vi "sql-readinfo-fixture.vi"(0 "input-IP":string="dg-sql-01.luxshare.com.cn", 1 "input-user":string="htpsuser", 3 "input-psw":string="htps'songyy", 4 "input-db":string="HTPSDB", 5 "操作模式":T1(ring)=enum."查询数据", 7 "查询项目":string="LuxsharePN,CustomerPN,Customer,SampleDes,AWG,Length,EEPROMWrite,LabelPrint,Remarks", 8 "表名":string="vfixture", 11 "标识列":string, 12 "限定条件":string="where LuxsharePN='L12345678'", 13 "Page":string, 15 "Desc":string) -> (14 "数据输出2":dbl[][](array[numeric]), 16 "错误类型":string, 17 "StringArray2":string[][](array[string])=[["L12345678\t\tIBM\t40G Ethernet QSFP+ Passive DAC Cable\t28\t3000\t0\t0\trefer to IBM Spec"]], 18 "列内对数":i32=1, 19 "返回记录数目":i32=1, 20 "ConvertToArray":string[][](array[string])=[["L12345678", "", "IBM", "40G Ethernet QSFP+ Passive DAC Cable", "28", "3000", "0", "0", "refer to IBM Spec"]], 21 "status":bool, 23 "ResultString":string="L12345678\t\tIBM\t40G Ethernet QSFP+ Passive DAC Cable\t28\t3000\t0\t0\trefer to IBM Spec\r", 24 "ConvertToClusterArray":cluster{"项":string, "值":string}[](array[cluster])=[{"项"="", "值"=""}, {"项"="L12345678", "值"="L12345678"}], 25 "DataPair":dbl[](array[numeric]), 27 "数据输出":dbl[][](array[numeric]))   [LabVIEW 2011]
panel:
  out "result string":string="select LuxsharePN,CustomerPN,Customer,SampleDes,AWG,Length,EEPROMWrite,LabelPrint,Remarks from project where LuxsharePN='L12345678'"
  out "替换数量":i32=9
  in  "二级分隔符":string
  in  "一级分隔符":string
  out "Result":bool=TRUE
  in  "InitArray1":string[][](array[string])
  in  "MoveToTail":i32=1
  in  "InitArray2":string[](array[string])
  out "错误输出":errorcluster
  in  "初始化簇数组":cluster{"项":string, "值":string}[](array[cluster])
  in  "簇元素":cluster{"项":string, "值":string}
  in  "ADODB._Recordset":refnum<k7>
  in  "ADODB._Connection":refnum<k7>
  # "列名 & 表名 查询结果"
  # "输       出"
  # "输       入"
  # "基本信息\n（）"
  # "状态灯，False表示操作成功，True表示操作失败"
  # "簇数组"
  # "限定条件，设定某个条件，输出满足该条件的数据"
  # "对数"
  # "错误类型"
  # "查询记录时才需要填写，page用于设置查询一次请求的记录数，Desc用于截断Desc条记录之前的记录"
  # "改变操作时需要修改的信息"
  # "操作模式：查询表名\n                  查询列名\n                  查询记录\n                  查询总记录\n                  查询数据"
  # "字符串"
  # "数组"
  # "查询表名时不需要输入\n\n查询列名和查询数据时要指定哪一张表"
  # "字符串数组"
  # "在查询表名和列名时不需要输入信息\n\n在查询数据时，如果要输入所有列，填入“*”，如果要查询指定的某一个列，输入该列的名称"
  # "ProjectName"
  # "EEPROMContent"
  # "LimitSpec"
  # "LabelContent"
  # "SwitchMatrix"
  # "error:\n-2147217843 登陆失败： 。\n-2147467259 要访问的数据库不存在\n-2146825267 没有数据    。\n-2146824584 对象关闭时，不允许操作\n-2147217865 表名不存在 。\n-2147467259 服务器连接失败 。"
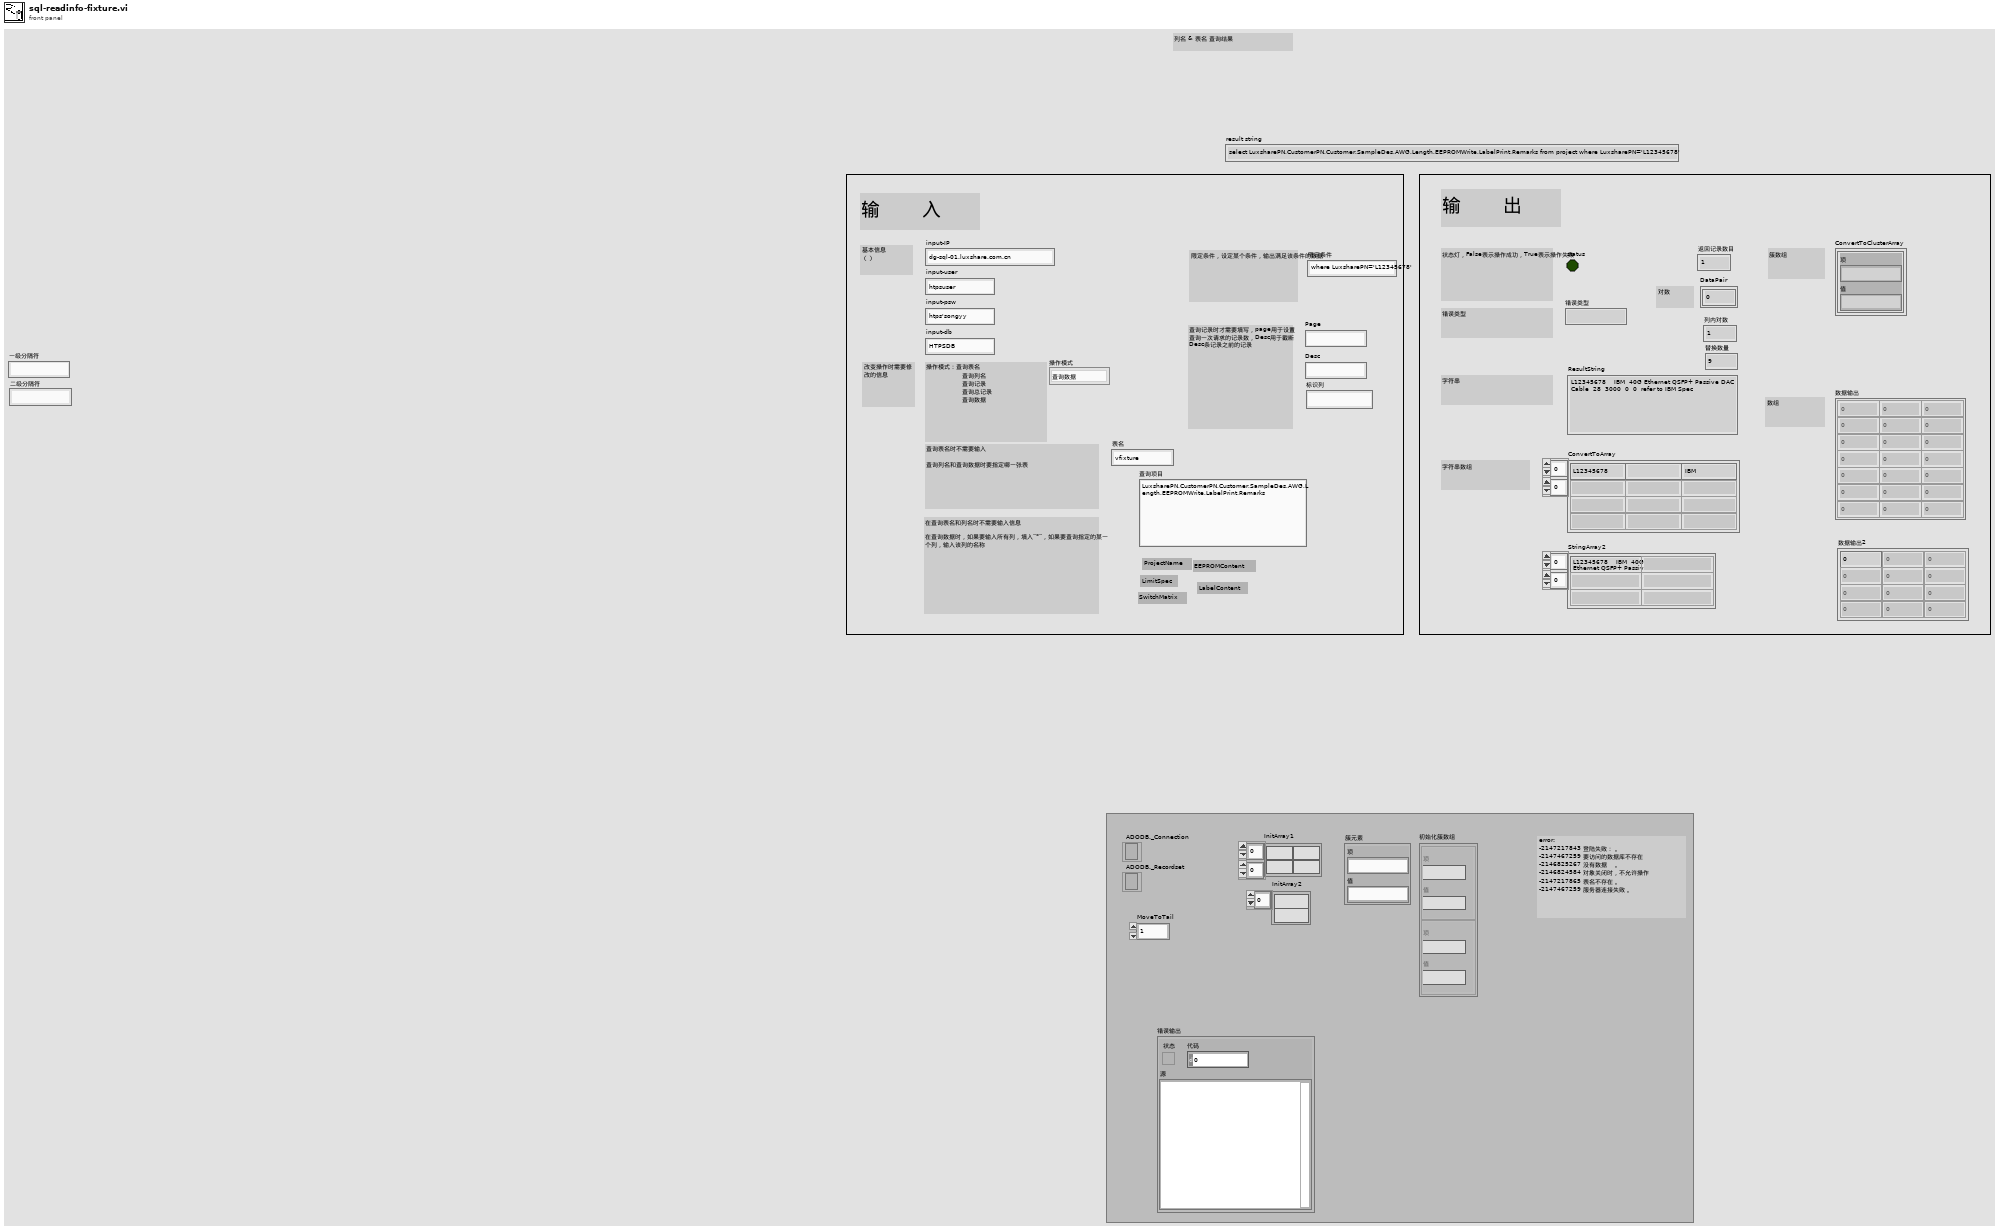
[diagram p1: front panel]
types:
  T1 = enum16{"查询表名", "查询列名", "查询记录", "查询总记录", "查询数据", "转换数据"}
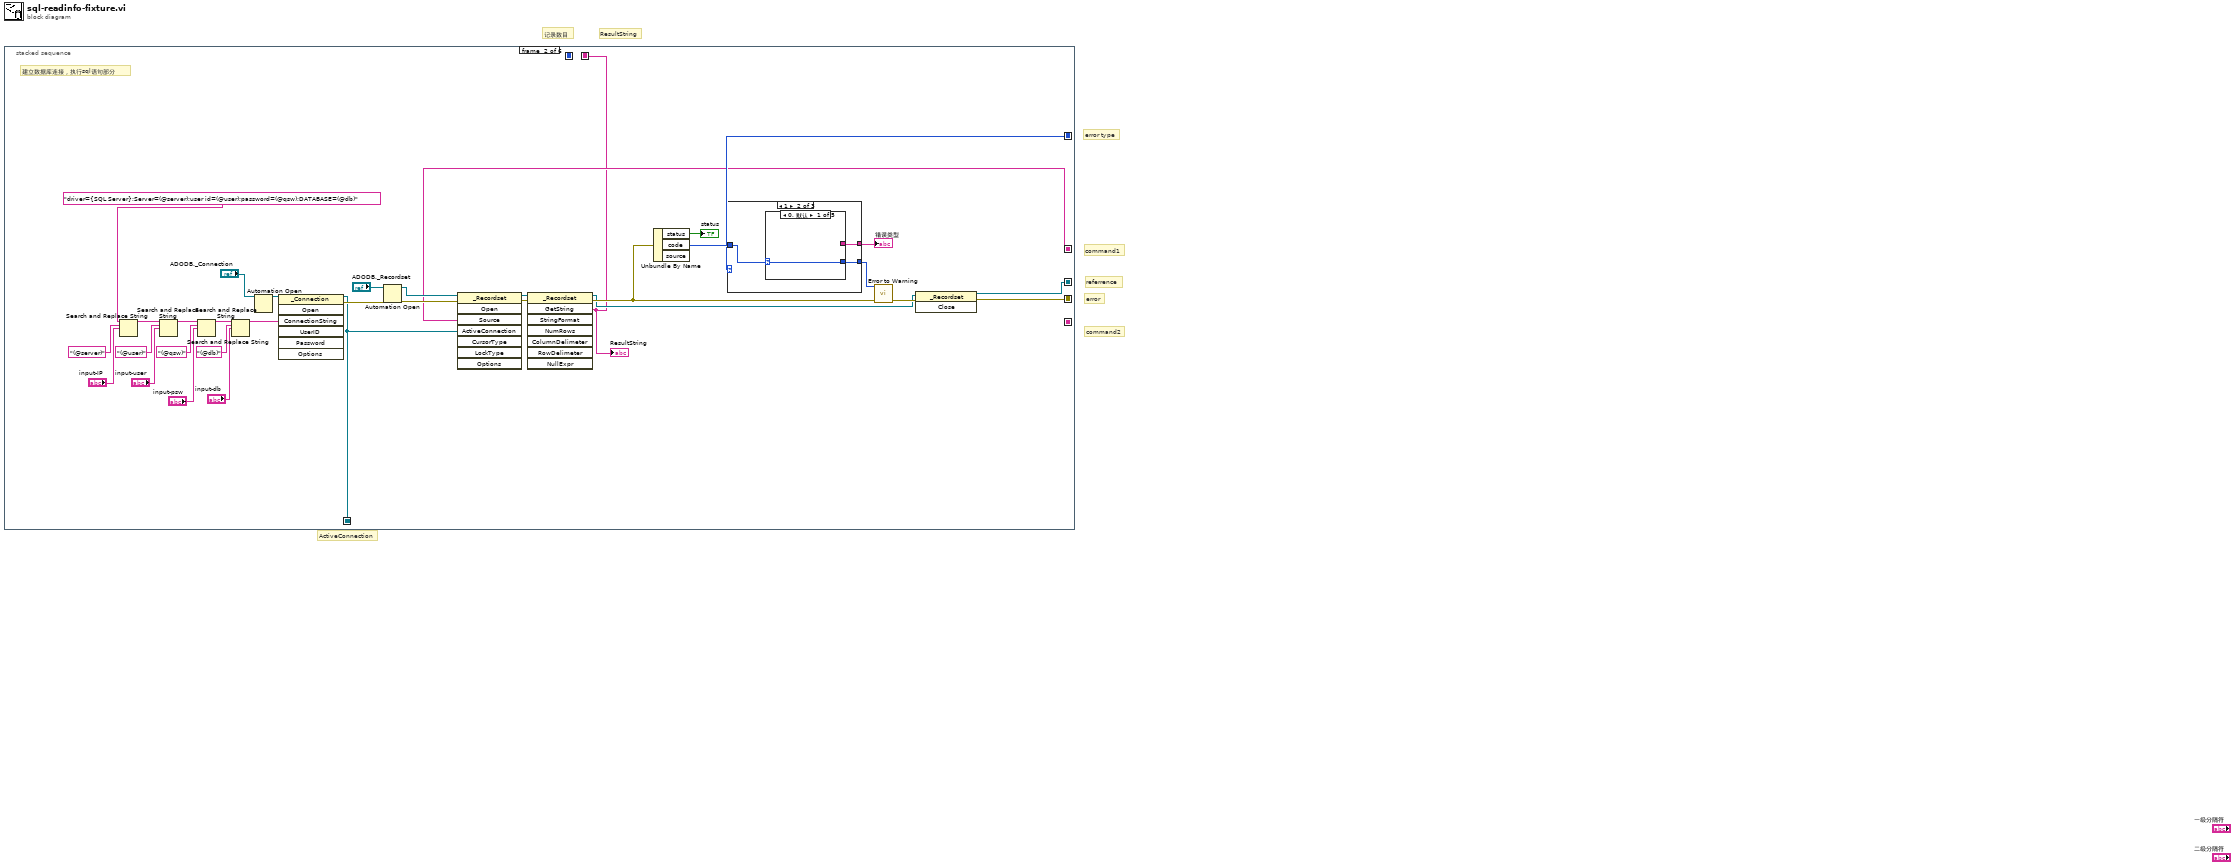
[diagram p0: block diagram]
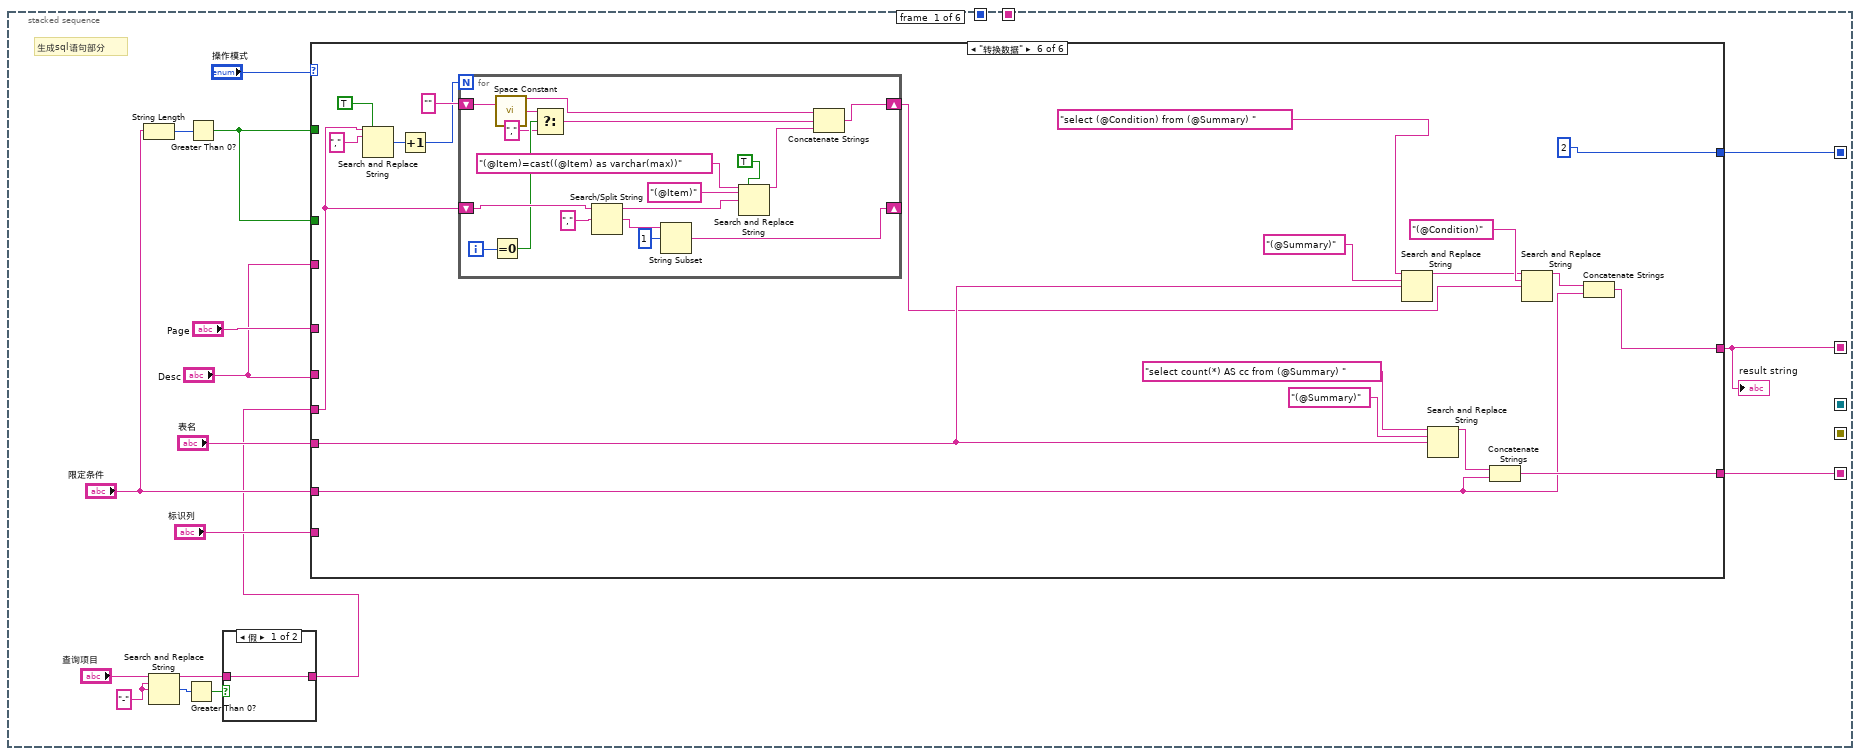
[diagram p2: hidden frame]
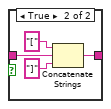
[diagram p3: hidden frame]
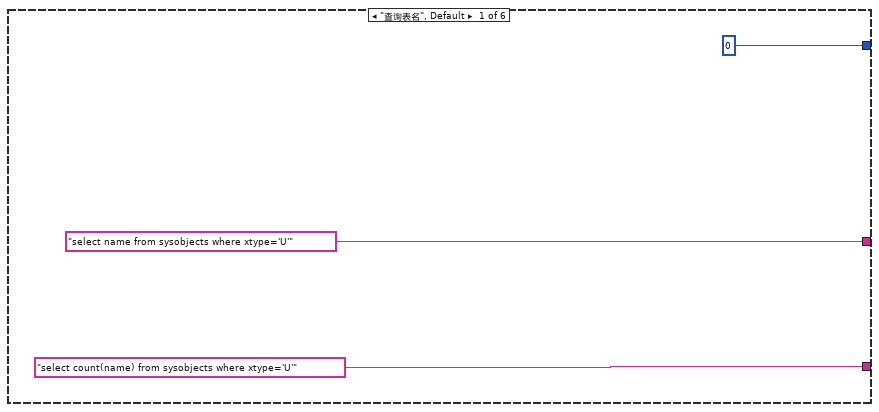
[diagram p4: hidden frame]
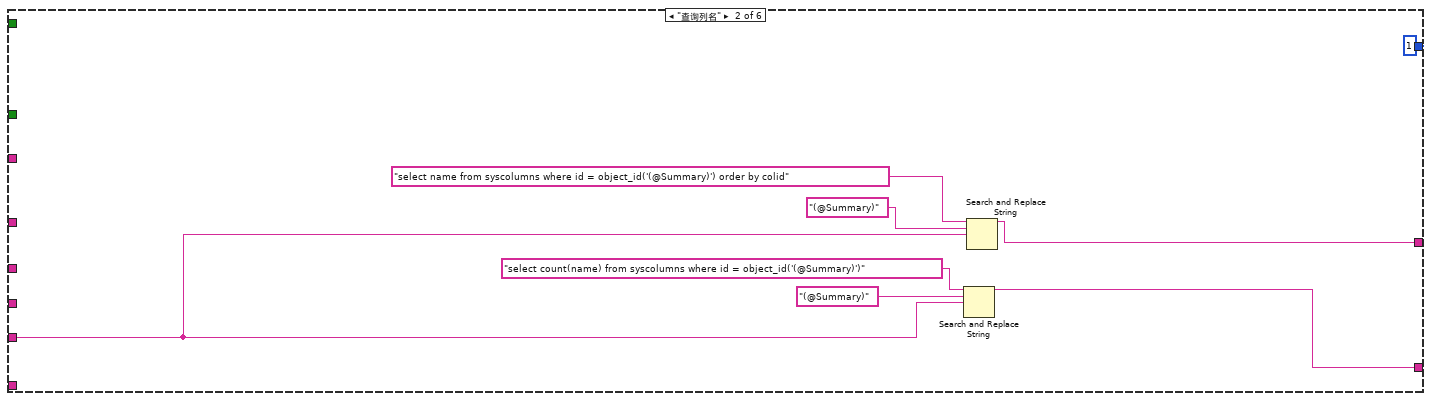
[diagram p5: hidden frame]
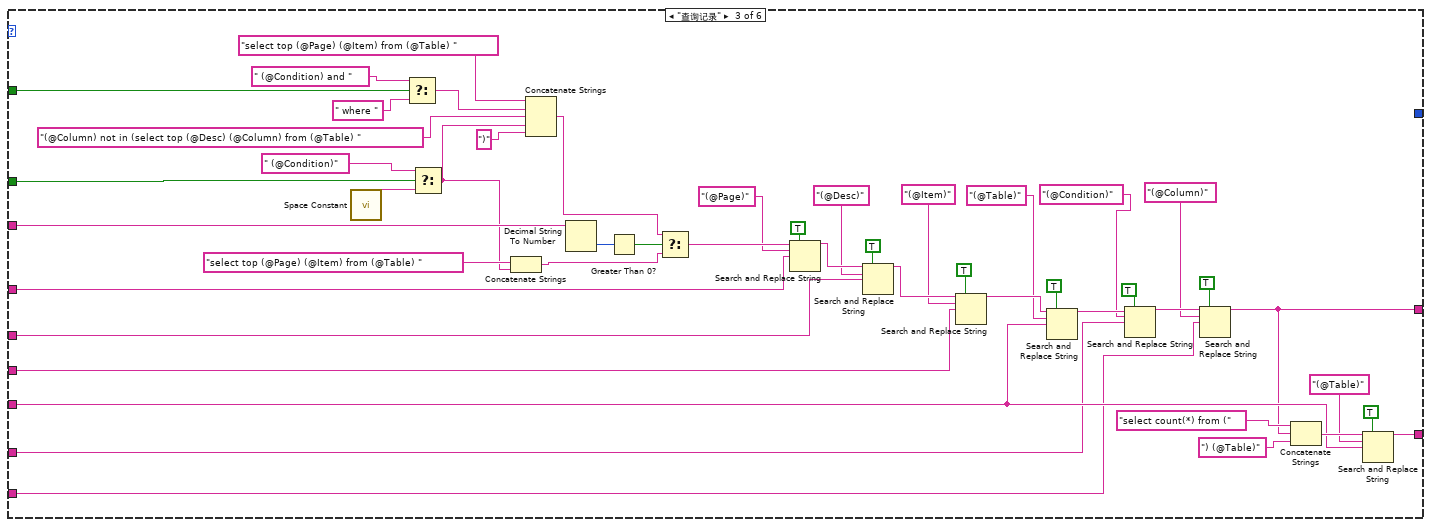
[diagram p6: hidden frame]
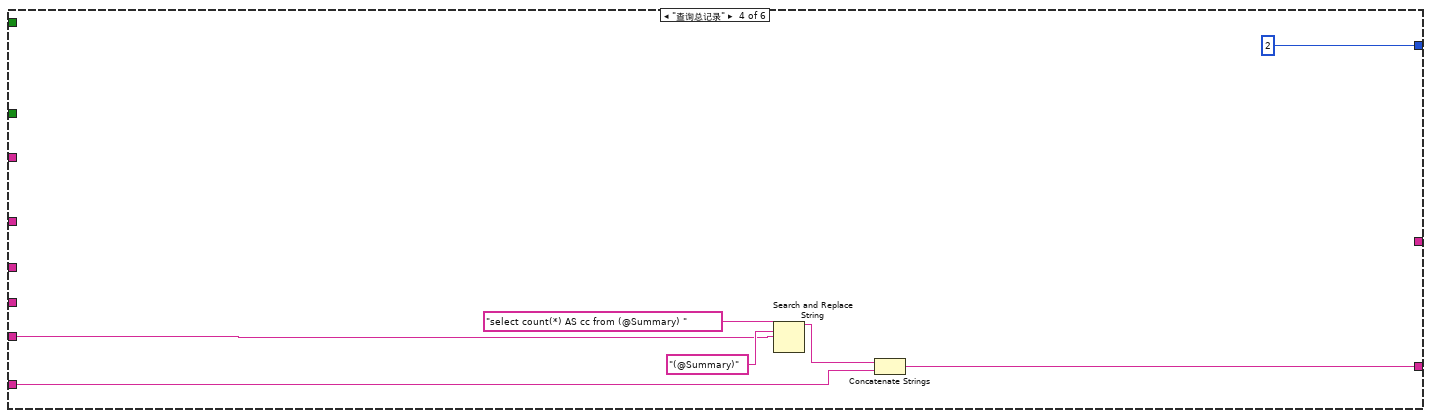
[diagram p7: hidden frame]
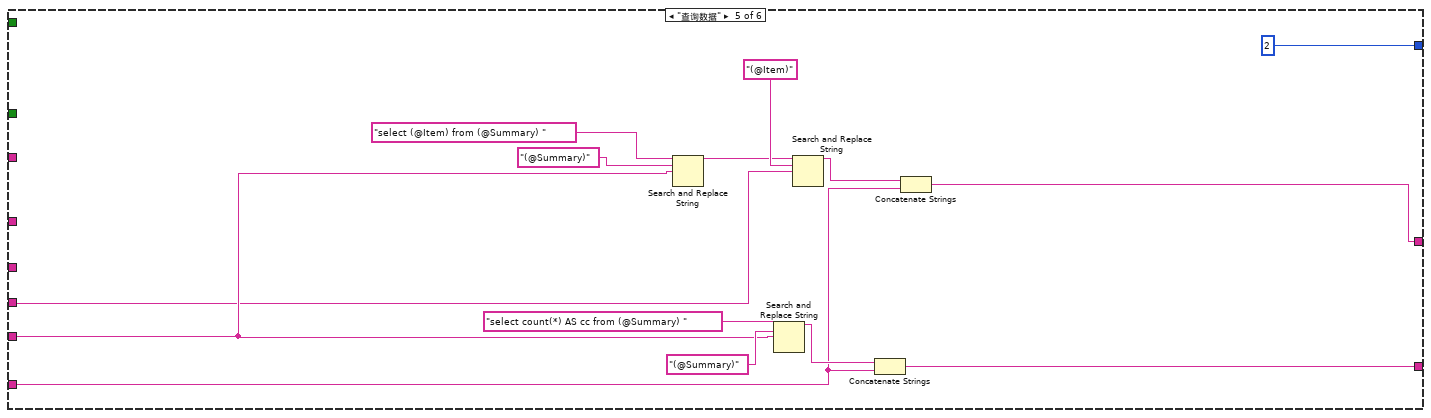
[diagram p8: hidden frame]
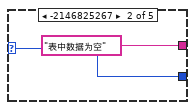
[diagram p10: hidden frame]
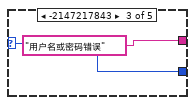
[diagram p11: hidden frame]
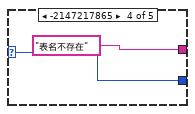
[diagram p12: hidden frame]
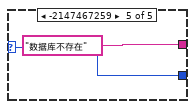
[diagram p13: hidden frame]
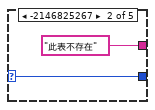
[diagram p14: hidden frame]
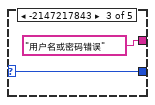
[diagram p15: hidden frame]
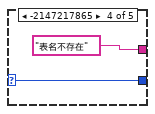
[diagram p16: hidden frame]
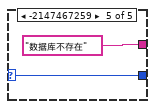
[diagram p17: hidden frame]
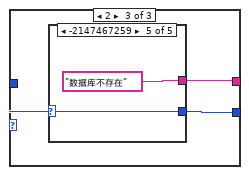
[diagram p18: hidden frame]
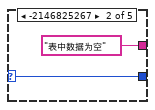
[diagram p20: hidden frame]
diagram:
  # "记录数目"
  # "ActiveConnection"
  # "referrence"
  # "error"
  # "error type"
  # "command2"
  # "command1"
  # "ResultString"
  n1 = stacked-sequence {
    seq-local: [_ w144 _ _ _ _] -> [_ _ w213 _ _ _]
    seq-local: [w5 _ _ _ _ _] -> [_ w146 _ _ _ _]
    seq-local: [w4 _ _ _ _ _] -> [_ w145 _ _ _ _]
    seq-local: [_ w143 _ _ _ _] -> [_ _ _ w234 w298 w354]
    seq-local: [_ w142 _ _ _ _] -> [_ _ w211 _ _ _]
    seq-local: [_ w141 _ _ _ _] -> [_ _ w212 _ _ _]
    seq-local: [w3 _ _ _ _ _] -> [_ _ w214 _ _ _]
    seq-local: [_ _ w210 _ _ _] -> [_ _ _ w235 _ _]
    frame #0 {
      w15 = "-"
      # "生成sql语句部分"
      n2 = String Length(string="限定条件") -> (length=w7:i32)
      n3 = Search and Replace String(input string="查询项目", search string=w15, replace string=w15) -> (result string=w12:string, number of replacements=w14:i32)  [unwired: 5 in, 2 out]
      n4 = Greater Than 0?(x=w14) -> (x > 0?=w13:bool)
      n5 = Greater Than 0?(x=w7) -> (x > 0?=w6:bool)
      n6 = case shown="假" w13 {
        tunnel: w12 -> [w18 w21]
        tunnel: [w18 w19] -> w1
        frame False {
        }
        frame True {
          n7 = Concatenate Strings("[", w21, "]") -> (w19:string)
        }
      }
      n8 = case shown="\"转换数据\"" "操作模式" {
        tunnel: "表名" -> [_ w30 w67 w86 w99 w111]
        tunnel: "限定条件" -> [_ _ w60 w83 w91 w114]
        tunnel: ["select name from sysobjects where xtype='U'" w28 w38 _ w92 w115] -> w4
        tunnel: ["select count(name) from sysobjects where xtype='U'" w29 w66 w84 w97 w119] -> w3
        tunnel: w1 -> [_ _ w72 _ w95 w104]
        tunnel: [0 1 _ 2 2 2] -> w5
        tunnel: "Page" -> [_ _ w79 _ _ _]
        tunnel: "Desc" -> [_ _ w78 _ _ _]
        tunnel: "Desc" -> [_ _ w58 _ _ _]
        tunnel: w6 -> [_ _ w54 _ _ _]
        tunnel: w6 -> [_ _ w50 _ _ _]
        tunnel: "标识列" -> [_ _ w34 _ _ _]
        frame "查询表名", Default {
        }
        frame "查询列名" {
          n9 = Search and Replace String(input string="select count(name) from syscolumns where id = object_id('(@Summary)')", search string="(@Summary)" ("搜索字符串"), replace string=w30) -> (result string=w29:string)  [unwired: 5 in, 3 out]
          n10 = Search and Replace String(input string="select name from syscolumns where id = object_id('(@Summary)') order by colid", search string="(@Summary)" ("搜索字符串"), replace string=w30) -> (result string=w28:string)  [unwired: 5 in, 3 out]
        }
        frame "查询记录" {
          n11 = call <vilib>:"Space Constant.vi"() -> ("String"=w51:string)
          n12 = Select(t=" (@Condition) and ", s=w54, f=" where ") -> (s? t:f=w48:string)
          n13 = Select(t=" (@Condition)", s=w50, f=w51) -> (s? t:f=w43:string)
          n14 = Concatenate Strings("select top (@Page) (@Item) from (@Table) ", w43) -> (w42:string)
          n15 = Concatenate Strings("select top (@Page) (@Item) from (@Table) ", w48, "(@Column) not in (select top (@Desc) (@Column) from (@Table) ", w43, ")") -> (w45:string)
          n16 = Decimal String To Number(string=w58) -> (number=w57:i32)  [unwired: 2 in, 1 out]
          n17 = Greater Than 0?(x=w57) -> (x > 0?=w56:bool)
          n18 = Select(t=w45, s=w56, f=w42) -> (s? t:f=w55:string)
          n19 = Search and Replace String(replace all?=TRUE ("替换全部？(F)"), input string=w55, search string="(@Page)" ("搜索字符串"), replace string=w79) -> (result string=w81:string)  [unwired: 4 in, 3 out]
          n20 = Search and Replace String(replace all?=TRUE ("替换全部？(F)"), input string=w81, search string="(@Desc)" ("搜索字符串"), replace string=w78) -> (result string=w75:string)  [unwired: 4 in, 3 out]
          n21 = Search and Replace String(replace all?=TRUE ("替换全部？(F)"), input string=w75, search string="(@Item)" ("搜索字符串"), replace string=w72) -> (result string=w70:string)  [unwired: 4 in, 3 out]
          n22 = Search and Replace String(replace all?=TRUE ("替换全部？(F)"), input string=w70, search string="(@Table)" ("搜索字符串"), replace string=w67) -> (result string=w62:string)  [unwired: 4 in, 3 out]
          n23 = Search and Replace String(replace all?=TRUE ("替换全部？(F)"), input string=w62, search string="(@Condition)" ("搜索字符串"), replace string=w60) -> (result string=w37:string)  [unwired: 4 in, 3 out]
          n24 = Search and Replace String(replace all?=TRUE ("替换全部？(F)"), input string=w37, search string="(@Column)" ("搜索字符串"), replace string=w34) -> (result string=w38:string)  [unwired: 4 in, 3 out]
          n25 = Concatenate Strings("select count(*) from (", w38, ") (@Table)") -> (w69:string)
          n26 = Search and Replace String(replace all?=TRUE ("替换全部？(F)"), input string=w69, search string="(@Table)" ("搜索字符串"), replace string=w67) -> (result string=w66:string)  [unwired: 4 in, 3 out]
        }
        frame "查询总记录" {
          n27 = Search and Replace String(input string="select count(*) AS cc from (@Summary) ", search string="(@Summary)" ("搜索字符串"), replace string=w86) -> (result string=w85:string)  [unwired: 5 in, 3 out]
          n28 = Concatenate Strings(w85, w83) -> (w84:string)
        }
        frame "查询数据" {
          n29 = Search and Replace String(input string="select (@Item) from (@Summary) ", search string="(@Summary)" ("搜索字符串"), replace string=w99) -> (result string=w93:string)  [unwired: 5 in, 3 out]
          n30 = Search and Replace String(input string="select count(*) AS cc from (@Summary) ", search string="(@Summary)" ("搜索字符串"), replace string=w99) -> (result string=w98:string)  [unwired: 5 in, 3 out]
          n31 = Search and Replace String(input string=w93, search string="(@Item)" ("搜索字符串"), replace string=w95) -> (result string=w94:string)  [unwired: 5 in, 3 out]
          n32 = Concatenate Strings(w98, w91) -> (w97:string)
          n33 = Concatenate Strings(w94, w91) -> (w92:string)
        }
        frame "转换数据" {
          n34 = Search and Replace String(replace all?=TRUE ("替换全部？(F)"), input string=w104, search string="," ("搜索字符串")) -> (number of replacements=w107:i32)  [unwired: 5 in, 3 out]
          n35 = Increment(x=w107) -> (x+1=w108:i32)
          n36 = for {
            N: w108 -> [_]
            shift-right: [w126] -> w105
            shift-left: "" -> [w127]
            shift-right: [w123] -> _
            shift-left: w104 -> [w138]
            i -> [w133]
            n37 = Equal To 0?(x=w133) -> (x = 0?=w132:bool)
            n38 = call <vilib>:"Space Constant.vi"() -> ("String"=w131:string)
            n39 = Select(t=w131, s=w132, f=",") -> (s? t:f=w129:string)
            n40 = Search/Split String(string=w138, search string/char (-)="," ("搜索字符串/字符(-)")) -> (substring before match=w135:string, match + rest of string=w125:string)  [unwired: 1 in, 1 out]
            n41 = String Subset(string=w125, offset (0)=1 ("偏移量(0)")) -> (substring=w123:string)  [unwired: 1 in]
            n42 = Search and Replace String(replace all?=TRUE ("替换全部？(F)"), input string="(@Item)=cast((@Item) as varchar(max))", search string="(@Item)", replace string=w135) -> (result string=w128:string)  [unwired: 4 in, 3 out]
            n43 = Concatenate Strings(w127, w129, w128) -> (w126:string)
          }
          n44 = Search and Replace String(input string="select (@Condition) from (@Summary) ", search string="(@Summary)" ("搜索字符串"), replace string=w111) -> (result string=w116:string)  [unwired: 5 in, 3 out]
          n45 = Search and Replace String(input string="select count(*) AS cc from (@Summary) ", search string="(@Summary)" ("搜索字符串"), replace string=w111) -> (result string=w120:string)  [unwired: 5 in, 3 out]
          n46 = Concatenate Strings(w120, w114) -> (w119:string)
          n47 = Search and Replace String(input string=w116, search string="(@Condition)" ("搜索字符串"), replace string=w105) -> (result string=w117:string)  [unwired: 5 in, 3 out]
          n48 = Concatenate Strings(w117, w114) -> (w115:string)
        }
      }
      "result string" <- w4
    }
    frame #1 {
      # "建立数据库连接，执行sql语句部分"
      n49 = Search and Replace String(input string="driver={SQL Server};Server=(@server);user id=(@user);password=(@qsw);DATABASE=(@db)" ("ConnectionString"), search string="(@server)" ("搜索字符串"), replace string="input-IP") -> (result string=w151:string)  [unwired: 5 in, 3 out]
      n50 = Search and Replace String(input string=w151, search string="(@user)" ("搜索字符串"), replace string="input-user") -> (result string=w154:string)  [unwired: 5 in, 3 out]
      n51 = Search and Replace String(input string=w154, search string="(@qsw)" ("搜索字符串"), replace string="input-psw") -> (result string=w157:string)  [unwired: 5 in, 3 out]
      n52 = Search and Replace String(input string=w157, search string="(@db)" ("搜索字符串"), replace string="input-db") -> (result string=w140:string)  [unwired: 5 in, 3 out]
      n53 = Automation Open(Automation Refnum="ADODB._Connection") -> (Automation Refnum=w147:refnum<k7>)  [unwired: 3 in, 1 out]
      n54 = invoke class="_Connection" method="Open"(reference=w147, "ConnectionString"=w140) -> (reference out=w144:refnum<k7>, error out=w163:errorcluster)  [unwired: 5 in, 5 out]
      n55 = Automation Open(error in (no error)=w163, Automation Refnum="ADODB._Recordset") -> (Automation Refnum=w162:refnum<k7>, error out=w164:errorcluster)  [unwired: 2 in]
      n56 = invoke class="_Recordset" method="Open"(reference=w162, error in=w164, "Source"=w145, "ActiveConnection"=w144) -> (reference out=w165:refnum<k7>, error out=w166:errorcluster)  [unwired: 4 in, 6 out]
      n57 = invoke class="_Recordset" method="GetString"(reference=w165, error in=w166) -> (reference out=w167:refnum<k7>, error out=w173:errorcluster, "GetString"=w143:string)  [unwired: 6 in, 5 out]
      "ResultString" <- w143
      n58 = Unbundle By Name(w173) -> ("status"=→"status":bool, "code"=w170:i32)  [unwired: 1 out]
      n59 = case shown="1" w146 {
        tunnel: w170 -> [w176 w188 w198]
        tunnel: [w175 w187 w200] -> w171
        tunnel: [w174 w186 w199] -> w172
        frame 0, Default {
          n60 = case shown="0, 默认" w176 {
            selector: w176 -> [w177 w179 w180 w183 w184]
            tunnel: [w177 w179 w180 w183 w184] -> w175
            tunnel: [_ "表中数据为空" "用户名或密码错误" "表名不存在" "数据库不存在"] -> w174
            frame 0, Default {
            }
            frame -2146825267 {
            }
            frame -2147217843 {
            }
            frame -2147217865 {
            }
            frame -2147467259 {
            }
          }
        }
        frame 1 {
          n61 = case shown="0, 默认" w188 {
            selector: w188 -> [w189 w191 w192 w195 w196]
            tunnel: [w189 w191 w192 w195 w196] -> w187
            tunnel: [_ "此表不存在" "用户名或密码错误" "表名不存在" "数据库不存在"] -> w186
            frame 0, Default {
            }
            frame -2146825267 {
            }
            frame -2147217843 {
            }
            frame -2147217865 {
            }
            frame -2147467259 {
            }
          }
        }
        frame 2 {
          n62 = case shown="-2147467259" w198 {
            selector: w198 -> [w201 w203 w204 w207 w208]
            tunnel: [w201 w203 w204 w207 w208] -> w200
            tunnel: [_ "表中数据为空" "用户名或密码错误" "表名不存在" "数据库不存在"] -> w199
            frame 0, Default {
            }
            frame -2146825267 {
            }
            frame -2147217843 {
            }
            frame -2147217865 {
            }
            frame -2147467259 {
            }
          }
        }
      }
      "错误类型" <- w172
      n63 = call <vilib>:"Error to Warning.vi"("1st Error to Convert"=w171, "error in"=w173) -> ("warning out"=w168:errorcluster)  [unwired: 13 in]
      n64 = invoke class="_Recordset" method="Close"(reference=w167, error in=w168) -> (reference out=w141:refnum<k7>, error out=w142:errorcluster)  [unwired: 1 in, 1 out]
    }
    frame #2 {
      # "执行sql语句部分\n此部分执行的sql语句的作用是统计返回的记录数目"
      n65 = call <vilib>:"Error to Warning.vi"("1st Error to Convert"=-2146824584, "error in"=w211) -> ("warning out"=w224:errorcluster)  [unwired: 13 in]
      n66 = invoke class="_Recordset" method="Open"(reference=w212, error in=w224, "Source"=w214, "ActiveConnection"=w213) -> (reference out=w219:refnum<k7>, error out=w223:errorcluster)  [unwired: 4 in, 6 out]
      n67 = invoke class="_Recordset" method="GetString"(reference=w219, error in=w223) -> (reference out=w221:refnum<k7>, error out=w226:errorcluster, "GetString"=w220:string)  [unwired: 6 in, 5 out]
      n68 = Decimal String To Number(string=w220) -> (number=w210:i32)  [unwired: 2 in, 1 out]
      "返回记录数目" <- w210
      n69 = call <vilib>:"Error to Warning.vi"("1st Error to Convert"=-2147217865, "error in"=w226) -> ("warning out"=w227:errorcluster)  [unwired: 13 in]
      n70 = Greater Than 0?(x=w210) -> (x > 0?=w215:bool)
      n71 = invoke class="_Recordset" method="Close"(reference=w221, error in=w227) -> (reference out=w222:refnum<k7>, error out=w230:errorcluster)  [unwired: 1 in, 1 out]
      n72 = Select(t=TRUE, s=w215, f=FALSE) -> (s? t:f=→"Result":bool)
      n73 = call <vilib>:"Error to Warning.vi"("1st Error to Convert"=-2147217864, "2nd Error to Convert"=-2147467259, "error in"=w230) -> ("warning out"=w231:errorcluster)  [unwired: 12 in]
      n74 = Close Reference(reference=w222, error in (no error)=w231) -> (error out=→"错误输出":errorcluster)
    }
    frame #3 {
      w250 = "\t"
      # "此部分对数据的处理主要针对记录"
      n75 = Search/Split String(string=w234, search string/char (-)="\r") -> (substring before match=w249:string)  [unwired: 1 in, 2 out]
      n76 = Search and Replace String(replace all?=TRUE ("替换全部？(F)"), input string=w249, search string=w250, replace string=w250) -> (number of replacements=w252:i32)  [unwired: 4 in, 3 out]
      n77 = Increment(x=w252) -> (x+1=w253:i32)
      "替换数量" <- w253
      n78 = for {
        N: w235 -> [_]
        shift-right: [w259] -> w246
        shift-left: "InitArray1" -> [w260]
        shift-right: [w256] -> _
        shift-left: w234 -> [w262]
        tunnel: w253 -> [w255]
        i -> [w257]
        n79 = Decrement(x=w255) -> (x-1=w254:i32)
        n80 = for {
          N: w255 -> [_]
          shift-right: [w271] -> w256
          shift-left: w262 -> [w275]
          shift-right: [w272] -> w258
          shift-left: "InitArray2" -> [w274]
          tunnel: w254 -> [w263]
          i -> [w268]
          n81 = Equal?(x=w268, y=w263) -> (x = y?=w267:bool)
          n82 = Select(t="return", s=w267, f="table") -> (s? t:f=w264:string)
          n83 = case shown="\"return\"" w264 {
            tunnel: ["," "" "\t" "\r" "\n" "\r\n"] -> w276
            frame "comma", Default {
            }
            frame "space" {
            }
            frame "table" {
              # "\\t"
            }
            frame "return" {
              # "\\r"
            }
            frame "newline" {
              # "\\n"
            }
            frame "lineover" {
              # "\\r\\n"
            }
          }
          n84 = Search/Split String(string=w275, search string/char (-)=w276) -> (substring before match=w273:string, match + rest of string=w270:string)  [unwired: 1 in, 1 out]
          n85 = Insert Into Array(array=w274, index=w268, new element=w273) -> (w272:string[])
          n86 = case shown="1, 默认" "MoveToTail" {
            tunnel: [w277 w279 w283] -> w271
            tunnel: w270 -> [w278 w280 w282]
            frame 1, Default {
              n87 = Rotate String(1:w278) -> (0:w277:string)
            }
            frame 2 {
              n88 = Rotate String(1:w280) -> (0:w281:string)
              n89 = Rotate String(1:w281) -> (0:w279:string)
            }
            frame 3 {
              n90 = Rotate String(1:w282) -> (0:w285:string)
              n91 = Rotate String(1:w285) -> (0:w284:string)
              n92 = Rotate String(1:w284) -> (0:w283:string)
            }
          }
        }
        n93 = Insert Into Array(array=w260, index (row)=w257, new element=w258) -> (w259:string[][])  [unwired: 1 in]
      }
      "ConvertToArray" <- w246
      n94 = Index Array(array=w246, index (col)=0 ("禁用的索引 (列)")) -> (element=w243:string[])  [unwired: 1 in]
      n95 = Array Size(array=w246) -> (size(s)=w239:i32[])
      n96 = Build Array (concatenate)("", w243) -> (w244:string[])
      n97 = Index Array(array=w239, index=0 ("索引")) -> (element=w241:i32)
      n98 = Increment(x=w241) -> (x+1=w247:i32)
      n99 = for {
        N: w247 -> [_]
        tunnel: w244 -> [w297] mode=indexing
        shift-right: [w294] -> w237
        shift-left: "初始化簇数组" -> [w295]
        i -> [w296]
        n100 = Bundle By Name(cluster="簇元素", "项"=w297, "值"=w297) -> (w292:cluster{"项":string, "值":string})
        n101 = Insert Into Array(array=w295, index=w296, new element=w292) -> (w294:cluster{"项":string, "值":string}[])
      }
      "ConvertToClusterArray" <- w237
    }
    frame #4 {
      w299 = ":" ("搜索字符串")
      # "此部分对数据处理针对具体的测量数据"
      n102 = Search and Replace String(replace all?=TRUE ("替换全部？(F)"), input string=w298, search string=w299, replace string=w299) -> (number of replacements=w301:i32)  [unwired: 4 in, 3 out]
      n103 = Increment(x=w301) -> (x+1=w306:i32)
      "列内对数" <- w306
      n104 = for {
        N: w306 -> [_]
        shift-right: [w315] -> _
        shift-left: w298 -> [w316]
        shift-right: [w313] -> w303
        shift-left: dbl[][] [] -> [w309]
        shift-right: [w307] -> w305
        shift-left: dbl[][] [] -> [w308]
        i -> [w312]
        n105 = while {
          shift-right: [w328] -> w310
          shift-left: dbl[] [] -> [w329]
          shift-right: [w330] -> w315
          shift-left: w316 -> [w331]
          i -> [w327]
          stop <- w325 stop-if-true
          n106 = while {
            shift-right: [w340] -> w330
            shift-left: w331 -> [w342]
            shift-right: [w338] -> w323
            shift-left: "" -> [w339]
            tunnel: [w336] -> w326
            stop <- w337 stop-if-true
            n107 = Search/Split String(string=w342, offset (0)=1 ("偏移量(0)")) -> (substring before match=w336:string, match + rest of string=w340:string)  [unwired: 1 in, 1 out]
            n108 = case shown="默认" w336 {
              selector: w336 -> [_ _ _ w351]
              tunnel: w339 -> [w343 w345 w348 w352]
              tunnel: [w343 w345 w348 w350] -> w338
              tunnel: [TRUE TRUE TRUE FALSE] -> w337
              frame ":" {
              }
              frame "," {
              }
              frame "" {
              }
              frame Default {
                n109 = Concatenate Strings(w352, w351) -> (w350:string)
              }
            }
          }
          n110 = Fract/Exp String To Number(string=w323) -> (number=w322:dbl)  [unwired: 3 in, 1 out]
          n111 = case shown="\",\"" w326 {
            tunnel: [TRUE FALSE TRUE TRUE] -> w325
            frame ":" {
            }
            frame "," {
            }
            frame "" {
            }
            frame Default {
            }
          }
          n112 = Insert Into Array(array=w329, index=w327, new element=w322) -> (w328:dbl[])
        }
        n113 = Greater Than 0?(x=w312) -> (x > 0?=w311:bool)
        n114 = case shown="真" w311 {
          tunnel: [w318 w321] -> w313
          tunnel: w309 -> [w318 w320]
          tunnel: w310 -> [w317 w319]
          frame False {
            "DataPair" <- w317
          }
          frame True {
            n115 = Insert Into Array(array=w320, new element=w319) -> (w321:dbl[][])  [unwired: 2 in]
          }
        }
        n116 = Insert Into Array(array=w308, new element=w310) -> (w307:dbl[][])  [unwired: 2 in]
      }
      "数据输出" <- w303
      "数据输出2" <- w305
    }
    frame #5 {
      (unwired) 0.0
      w355 = ":" ("搜索字符串")
      # "此部分对数据处理针对具体的测量数据"
      n117 = Search and Replace String(replace all?=TRUE ("替换全部？(F)"), input string=w354, search string=w355, replace string=w355) -> (number of replacements=w357:i32)  [unwired: 4 in, 3 out]
      n118 = Increment(x=w357) -> (x+1=w359:i32)
      n119 = for {
        N: w359 -> [_]
        shift-right: [w365] -> _
        shift-left: w354 -> [w366]
        shift-right: [w360] -> w353
        shift-left: string[][] [] -> [w361]
        i -> [w363]
        n120 = Greater Than 0?(x=w363) -> ()  [unwired: 1 out]
        n121 = while {
          shift-right: [w373] -> w362
          shift-left: string[] [] -> [w374]
          shift-right: [w375] -> w365
          shift-left: w366 -> [w376]
          i -> [w372]
          stop <- w370 stop-if-true
          n122 = while {
            shift-right: [w385] -> w375
            shift-left: w376 -> [w387]
            shift-right: [w383] -> w368
            shift-left: "" -> [w384]
            tunnel: [w381] -> w371
            stop <- w382 stop-if-true
            n123 = Search/Split String(string=w387, offset (0)=1 ("偏移量(0)")) -> (substring before match=w381:string, match + rest of string=w385:string)  [unwired: 1 in, 1 out]
            n124 = case shown="\"\"" w381 {
              selector: w381 -> [_ _ _ w396]
              tunnel: w384 -> [w388 w390 w393 w397]
              tunnel: [w388 w390 w393 w395] -> w383
              tunnel: [TRUE TRUE TRUE FALSE] -> w382
              frame ":" {
              }
              frame "," {
              }
              frame "" {
              }
              frame Default {
                n125 = Concatenate Strings(w397, w396) -> (w395:string)
              }
            }
          }
          n126 = call <vilib>:"Trim Whitespace.vi"("string"=w368) -> ("trimmed string"=w367:string)  [unwired: 1 in]
          n127 = case shown="\",\"" w371 {
            tunnel: [TRUE FALSE TRUE TRUE] -> w370
            frame ":" {
            }
            frame "," {
            }
            frame "" {
            }
            frame Default {
            }
          }
          n128 = Insert Into Array(array=w374, index=w372, new element=w367) -> (w373:string[])
        }
        n129 = Insert Into Array(array=w361, new element=w362) -> (w360:string[][])  [unwired: 2 in]
      }
      "StringArray2" <- w353
    }
  }
